vi "Configure Trend Line.vi"(0 "VISA resource name":refnum<visa-resource-name>, 5 "Trend Line (2: Normal)":i32(ring)=2 items=["Thin"=1, "Normal"=2, "Thick"=3], 7 "Grid (0 : Auto)":i32(ring) items=["Auto"=0, "4"=4, "5"=5, "6"=6, "7"=7, "8"=8, "9"=9, "10"=10, "11"=11, "12"=12], 11 "error in (no error)":errorcluster) -> (4 "VISA resource name out":refnum<visa-resource-name>, 15 "error out":errorcluster)   [LabVIEW 2020, in "Yokogawa GX Series.lvlib"]
doc: "Sets the trend waveform line width and the grid in the display area.\n\nCommand: STrdLine\n\nNote: This VI does nothing when the instrument is GM10."
uses:
  <instrlib>/Yokogawa GX Series/Yokogawa GX Series.lvlib
panel:
  # "div"
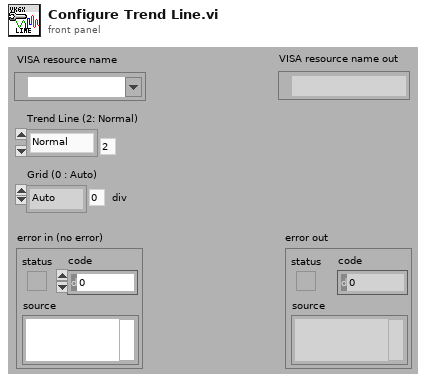
[diagram p1: front panel]
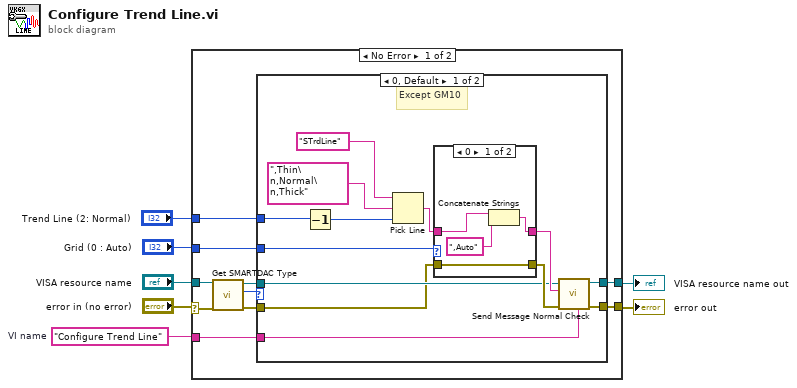
[diagram p0: block diagram]
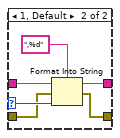
[diagram p2: hidden frame]
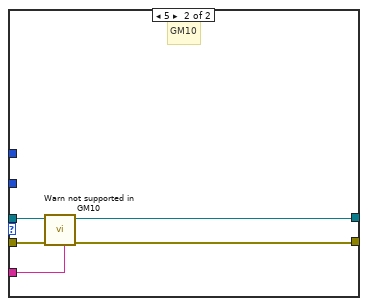
[diagram p3: hidden frame]
diagram:
  w3 = "Configure Trend Line"  # VI name
  n1 = case shown="No Error" "error in (no error)" {
    selector: "error in (no error)" -> [w11 w46]
    tunnel: "Trend Line (2: Normal)" -> [w14 _]
    tunnel: [w17 w47] -> w6
    tunnel: [w16 w46] -> w5
    tunnel: "Grid (0 : Auto)" -> [w13 _]
    tunnel: w3 -> [w15 _]
    tunnel: "VISA resource name" -> [w12 w47]
    frame No Error {
      n2 = call <instrlib>:"Get SMARTDAC Type.vi"("error in (no error)"=w11, "VISA resource name"=w12) -> ("error out"=w9:errorcluster, "SMARTDAC+ Type"=w8:u16, "VISA resource name out"=w10:refnum<visa-resource-name>)  [unwired: 7 in]
      n3 = case shown="0, Default" w8 {
        tunnel: [w30 w43] -> w17
        tunnel: [w29 w42] -> w16
        tunnel: w15 -> [w26 w41]
        tunnel: w14 -> [w25 _]
        tunnel: w13 -> [w23 _]
        tunnel: w10 -> [w19 w45]
        tunnel: w9 -> [w18 w44]
        frame 0, Default {
          # "Except GM10"
          n4 = Decrement(x=w25) -> (x-1=w24:i32)
          n5 = Pick Line(string ("")="STrdLine" ("形式文字列"), multi-line string=",Thin\n,Normal\n,Thick", line index=w24) -> (output string=w22:string)
          n6 = case shown="0" w23 {
            selector: w23 -> [_ w40]
            tunnel: w22 -> [w33 w38]
            tunnel: [w32 w36] -> w21
            tunnel: w18 -> [w31 w39]
            tunnel: [w31 w35] -> w20
            frame 0 {
              n7 = Concatenate Strings(w33, ",Auto") -> (w32:string)
            }
            frame 1, Default {
              n8 = Format Into String(format string=",%d", initial string=w38, error in=w39, w40) -> (resulting string=w36:string, error out=w35:errorcluster)
            }
          }
          n9 = call <instrlib>:"Send Message Normal Check.vi"("Source (\"\")"=w26, "error in (no error)"=w20, "Send Message (\"\")"=w21, "VISA resource name"=w19) -> ("error out"=w29:errorcluster, "VISA resource name out"=w30:refnum<visa-resource-name>)  [unwired: 2 in, 4 out]
        }
        frame 5 {
          # "GM10"
          n10 = call <instrlib>:"Warn not supported in GM10.vi"("Source (\"\")"=w41, "error in (no error)"=w44, "VISA resource name"=w45) -> ("error out"=w42:errorcluster, "VISA resource name out"=w43:refnum<visa-resource-name>)  [unwired: 7 in]
        }
      }
    }
    frame Error {
    }
  }
  "error out" <- w5
  "VISA resource name out" <- w6
